vi "Add to Array if Not Present (Path).vi"(4 "Path":path, 5 "String Array":path[](array[path])) -> (1 "New String Array":path[](array[path]))   [LabVIEW 2011]
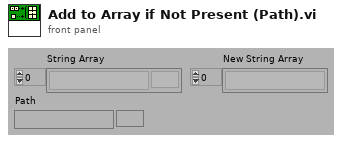
[diagram p1: front panel]
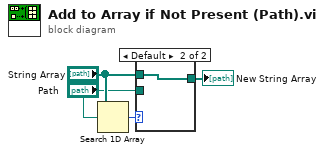
[diagram p0: block diagram]
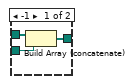
[diagram p2: hidden frame]
diagram:
  n1 = Search 1D Array(1D array="String Array", element="Path") -> (index of element=w4:i32)  [unwired: 1 out]
  n2 = case shown="Default" w4 {
    tunnel: "String Array" -> [w7 w8]
    tunnel: "Path" -> [w6 _]
    tunnel: [w5 w8] -> w1
    frame -1 {
      n3 = Build Array (concatenate)(w7, w6) -> (w5:path[])
    }
    frame Default {
    }
  }
  "New String Array" <- w1
